vi "DUAL GAUGE-RW Display control digits.vi"(7 "W/R":bool, 8 "Fehler (Eingang)":errorcluster, 9 "Displax control digits":i32(ring) items=["2 digits (default)", "3 digits"], 11 "Referenz in":refnum<visa-resource-name>) -> (0 "Cluster (Ausgang)":errorcluster, 1 "Get Display control digits":i32(ring) items=["2 digits", "3 digits"], 3 "Referenz out":refnum<visa-resource-name>)   [LabVIEW 2010, in "Dual Gauge.lvlib"]
uses:
  Dual Gauge.lvlib
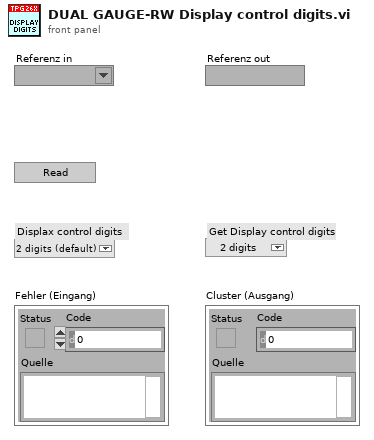
[diagram p1: front panel]
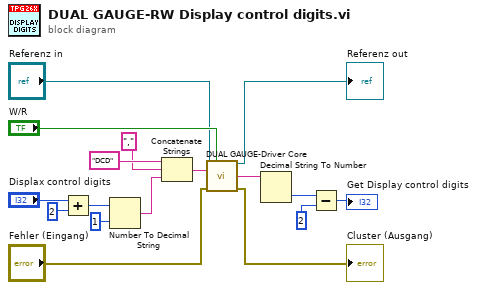
[diagram p0: block diagram]
diagram:
  n1 = Add(x="Displax control digits", y=i16 2 ("width (-)")) -> (x+y=w14:i32)
  n2 = Number To Decimal String(number=w14, width (-)=i16 1) -> (decimal integer string=w11:string)
  n3 = Concatenate Strings("DCD" ("Command"), "," ("Command"), w11) -> (w5:string)
  n4 = call "DUAL GAUGE-Driver Core.vi"("Referenz in"="Referenz in", "Write/Read"="W/R", "Command"=w5, "Fehler (Eingang)"="Fehler (Eingang)") -> ("Referenz out"=→"Referenz out":refnum<visa-resource-name>, "String Out"=w9:string, "Cluster (Ausgang)"=→"Cluster (Ausgang)":errorcluster)  [unwired: 9 in]
  n5 = Decimal String To Number(string=w9) -> (number=w7:i32)  [unwired: 2 in, 1 out]
  n6 = Subtract(x=w7, y=i16 2 ("width (-)")) -> (x-y=→"Get Display control digits":i32)
